vi "Kaiser-Bessel Window (CDB).vi"(2 "beta":dbl format="%0.2f", 3 "X":cdb[](array[numeric])) -> (0 "error":i32, 1 "Windowed X":cdb[](array[numeric]))   [LabVIEW 2010, in "NI_AALPro.lvlib"]
doc: "Applies a Kaiser-Bessel window to the input sequence <B>X</B>. Wire data to the <B>X</B> input to determine the polymorphic instance to use or manually select the instance."
uses:
  NI_AALPro.lvlib
  lvanlys.dll
panel:
  # "Kaiser-Bessel Window"
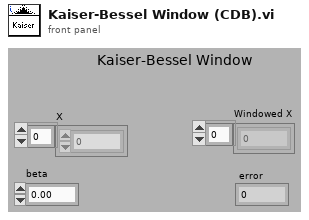
[diagram p1: front panel]
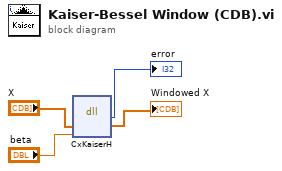
[diagram p0: block diagram]
diagram:
  n1 = dll-call lib="C:/Program Files/National Instruments/LabVIEW 2010/resource/lvanlys.*" fn="CxKaiserH"("X"="X", "beta"="beta") -> (→"error":i32, "X"=→"Windowed X":cdb[])  [unwired: 4 in, 2 out]
